vi "ProbeCerebellum.vi"(11 "Cerebellum out":refnum<class "Cerebellum.lvclass">) -> (2 "Value String":string, 3 "Boolean":bool)   [LabVIEW 2016, in "Cerebellum.lvclass"]
uses:
  Cerebellum/Cerebellum.lvclass
  Cerebellum/Cerebellum.lvclass/Cerebellum.ctl
  AER/AER.lvclass/AER.ctl
  AER/Get Currents.vi
  AER/Get No Neurons.vi
panel:
  out "No N":i32[](array[numeric])
  out "Firing Rate":cluster{"Numeric":dbl, "Numeric":dbl}(graph)
  in  "Neuron Left":i32
  in  "Neuron Righ":i32
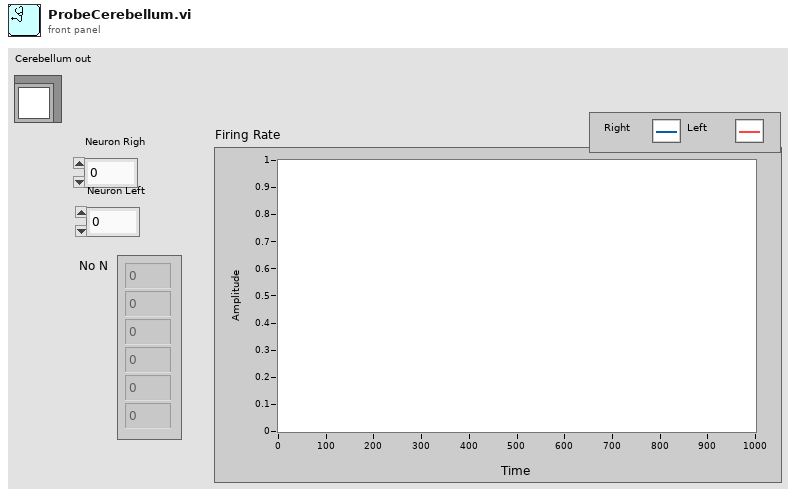
[diagram p1: front panel]
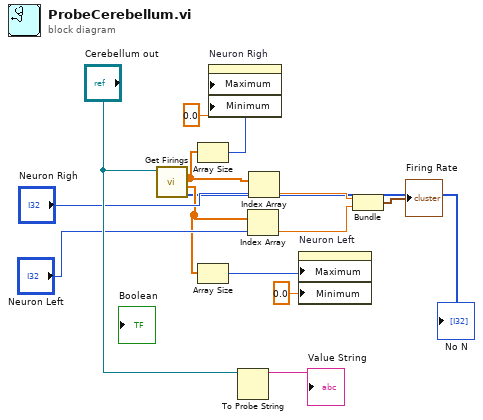
[diagram p0: block diagram]
diagram:
  n1 = call "Get Firings.vi"("Cerebellum in"="Cerebellum out") -> ("No N"=→"No N":i32[], "Currents Left"=w7:dbl[], "Currents Right"=w10:dbl[])  [unwired: 7 in, 1 out]
  n2 = Array Size(array=w10) -> (size(s)=w9:i32)
  n3 = Array Size(array=w7) -> (size(s)=w6:i32)
  n4 = property on="Neuron Righ" class="DigNum (strict)"("Maximum"=w9, "Minimum"=0.0 ("Data Entry Limits:Minimum")) -> ()  [unwired: 2 in, 2 out]
  n5 = To Probe String(7:"Cerebellum out") -> (3:→"Value String":string)  [unwired: 2 in, 1 out]
  n6 = Index Array(array=w7, index="Neuron Left") -> (element=w3:dbl)
  n7 = Index Array(array=w10, index="Neuron Righ") -> (element=w4:dbl)
  n8 = property on="Neuron Left" class="DigNum (strict)"("Maximum"=w6, "Minimum"=0.0 ("Data Entry Limits:Minimum")) -> ()  [unwired: 2 in, 2 out]
  n9 = Bundle("Numeric"=w4, "Numeric"=w3) -> (→"Firing Rate":cluster{"Numeric":dbl, "Numeric":dbl})  [unwired: 1 in]
